vi "Analyse.vi"(8 "error in (no error)":errorcluster, 10 "ImageData":T1, 11 "AbsorptionDS in":refnum<class "AbsorptionDS.lvclass">) -> (0 "error out":errorcluster, 3 "AbsorptionDS out":refnum<class "AbsorptionDS.lvclass">)   [LabVIEW 2009, in "Tools.lvlib" / "Imaging.lvlib" / "AbsorptionDS.lvclass"]
uses:
  AbsorptionDS.lvclass
  AbsorptionDS.lvclass/AbsorptionDS.ctl
  AbsorptionAnalyser/AbsorptionAnalyser.lvclass
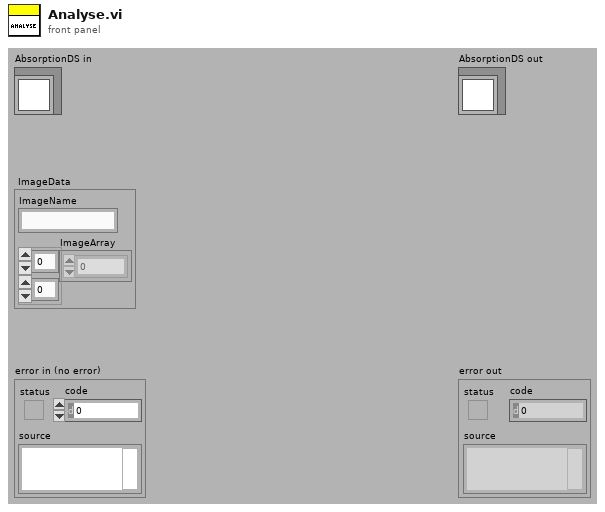
[diagram p1: front panel]
types:
  T1 = cluster{"ImageName":string, "ImageArray":sgl[][]}
  T2 = cluster{"ImageName":string, "ImageArray":sgl[][]}[]
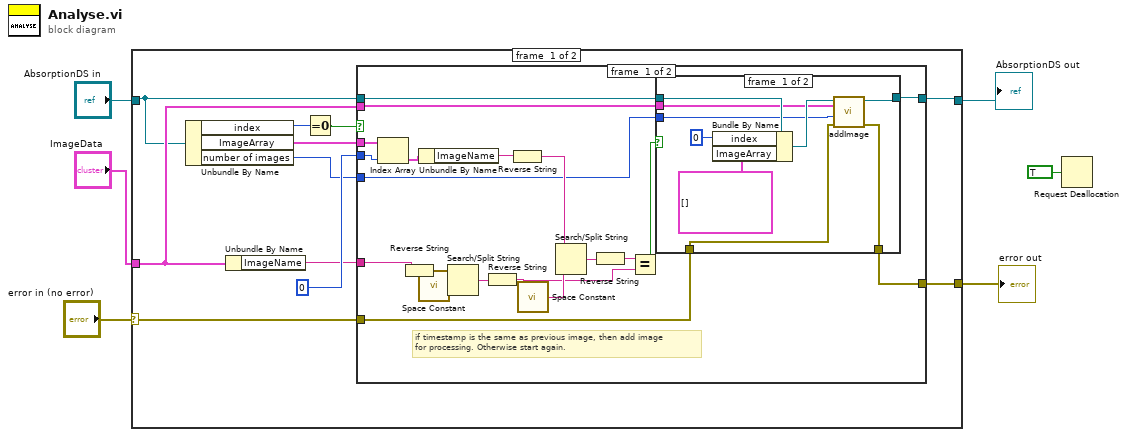
[diagram p0: block diagram]
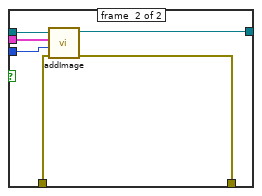
[diagram p2: hidden frame]
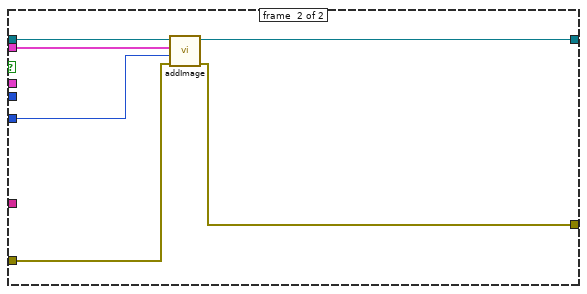
[diagram p3: hidden frame]
diagram:
  n1 = case shown="No Error" "error in (no error)" {
    selector: "error in (no error)" -> [w16 w59]
    tunnel: [w15 w59] -> w3
    tunnel: [w17 w60] -> w2
    tunnel: "AbsorptionDS in" -> [w7 w60]
    tunnel: "ImageData" -> [w14 _]
    frame #0 {
      n2 = Unbundle By Name(w7) -> ("index"=w10:i32, "ImageArray"=w13:T2, "number of images"=w8:i32)
      n3 = Unbundle By Name(w14) -> ("ImageName"=w9:string)
      n4 = Equal To 0?(x=w10) -> (x = 0?=w11:bool)
      n5 = case shown="True" w11 {
        tunnel: [w22 w58] -> w17
        tunnel: w16 -> [w20 w57]
        tunnel: [w19 w56] -> w15
        tunnel: w14 -> [w21 w55]
        tunnel: w7 -> [w23 w54]
        tunnel: w13 -> [w36 _]
        tunnel: 0 -> [w37 _]
        tunnel: w9 -> [w27 _]
        tunnel: w8 -> [w18 w53]
        frame #0 {
          # "if timestamp is the same as previous image, then add image\nfor processing. Otherwise start again."
          n6 = Index Array(array=w36, index=w37) -> (element=w35:T1)
          n7 = Reverse String(1:w27) -> (0:w30:string)
          n8 = Unbundle By Name(w35) -> ("ImageName"=w34:string)
          n9 = call <vilib>:"Space Constant.vi"() -> ("String"=w29:string)
          n10 = Search/Split String(string=w30, search string/char (-)=w29) -> (match + rest of string=w28:string)  [unwired: 1 in, 2 out]
          n11 = Reverse String(1:w28) -> (0:w25:string)
          n12 = Reverse String(1:w34) -> (0:w33:string)
          n13 = call <vilib>:"Space Constant.vi"() -> ("String"=w32:string)
          n14 = Search/Split String(string=w33, search string/char (-)=w32) -> (match + rest of string=w31:string)  [unwired: 1 in, 2 out]
          n15 = Reverse String(1:w31) -> (0:w26:string)
          n16 = Equal?(x=w26, y=w25) -> (x = y?=w24:bool)
          n17 = case shown="True" w24 {
            tunnel: w23 -> [w45 w52]
            tunnel: [w43 w51] -> w22
            tunnel: w21 -> [w41 w50]
            tunnel: w20 -> [w40 w49]
            tunnel: [w39 w48] -> w19
            tunnel: w18 -> [w38 w47]
            frame #0 {
              n18 = Bundle By Name(cluster=w45, "index"=0, "ImageArray"=T2 []) -> (w44:refnum<class "AbsorptionDS.lvclass">)
              n19 = call "addImage.vi"("error in (no error)"=w40, "number of images"=w38, "ImageData"=w41, "AbsorptionAnalyser in"=w44) -> ("error out"=w39:errorcluster, "AbsorptionAnalyser out"=w43:refnum<class "AbsorptionDS.lvclass">)  [unwired: 6 in]
            }
            frame #1 {
              n20 = call "addImage.vi"("error in (no error)"=w49, "number of images"=w47, "ImageData"=w50, "AbsorptionAnalyser in"=w52) -> ("error out"=w48:errorcluster, "AbsorptionAnalyser out"=w51:refnum<class "AbsorptionDS.lvclass">)  [unwired: 6 in]
            }
          }
        }
        frame #1 {
          n21 = call "addImage.vi"("error in (no error)"=w57, "number of images"=w53, "ImageData"=w55, "AbsorptionAnalyser in"=w54) -> ("error out"=w56:errorcluster, "AbsorptionAnalyser out"=w58:refnum<class "AbsorptionDS.lvclass">)  [unwired: 6 in]
        }
      }
    }
    frame #1 {
    }
  }
  "error out" <- w3
  "AbsorptionDS out" <- w2
  n22 = Request Deallocation(TRUE ("flag")) -> ()
